vi "Create or Access Config Path.vi"(8 "error in":errorcluster, 10 "Check/Build Folders?":bool, 11 "Module Data":refnum<class "Rename.lvclass">) -> (0 "error out":errorcluster, 2 "Config File Path":path, 3 "Module Data":refnum<class "Rename.lvclass">)   [LabVIEW 2015, in "Generic Module Library.lvlib" / "Template G_Module.lvlib"]
uses:
  Template G_Module.lvlib
  <vilib>/Utility/sysdir.llb/System Directory Type.ctl
  Module Class/Rename.lvclass
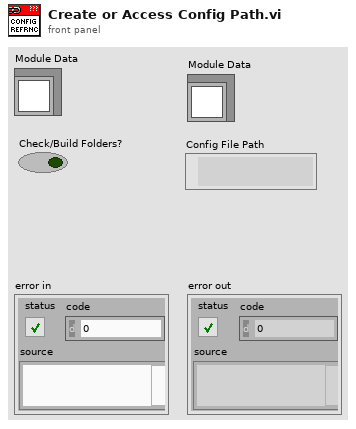
[diagram p1: front panel]
types:
  T1 = enum16{"open", "replace", "create", "open or create", "replace or create", "replace or create with confirmation"}
  T2 = typedef "System Directory Type.ctl" = i32
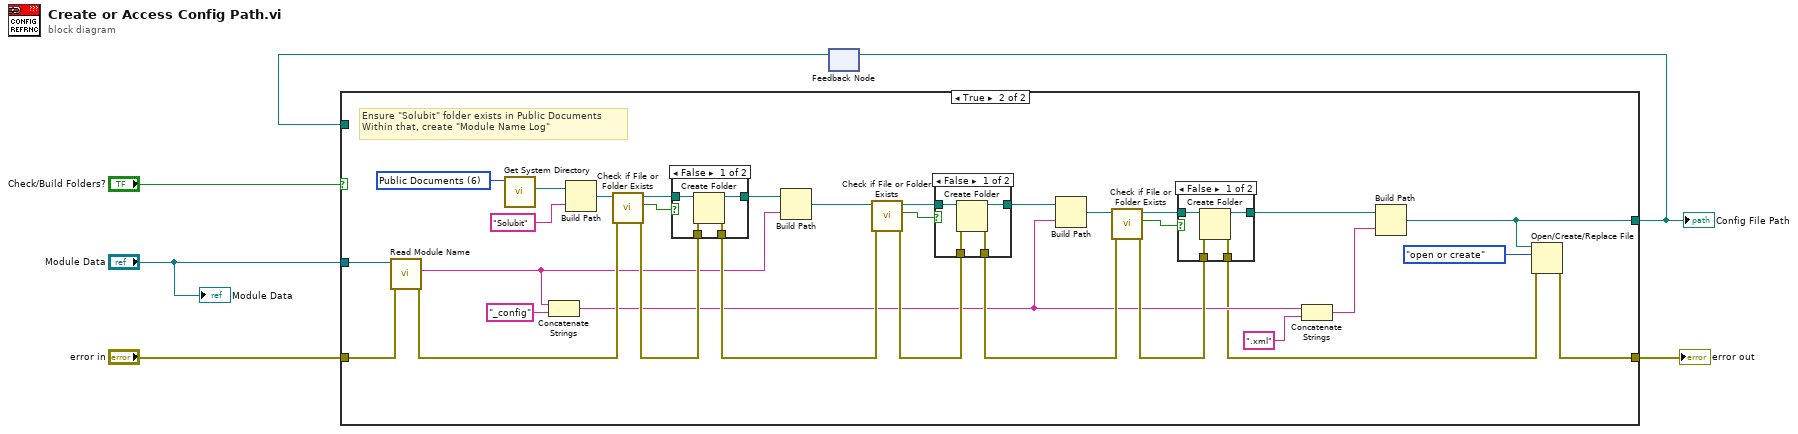
[diagram p0: block diagram]
diagram:
  n1 = feedback #1() -> (w2:path)  [unwired: 1 in]
  n2 = case shown="True" "Check/Build Folders?" {
    tunnel: "Module Data" -> [_ w33]
    tunnel: "error in" -> [w8 w32]
    tunnel: [w8 w10] -> w5
    tunnel: [w7 w12] -> w1
    tunnel: w2 -> [w7 _]
    frame False {
    }
    frame True {
      w40 = T2 6 items=["User Home"=0, "User Desktop"=1, "User Documents"=2, "User Application Data"=3, "User Preferences"=4, "User Temporary"=5, "Public Documents"=6, "Public Application Data"=7, "Public Preferences"=8, "Public Cache"=13, "System Core Libraries"=9, "System Installed Libraries"=10, "Application Files"=11, "Boot Volume Root"=12] ("system directory type")
      # "Ensure \"Solubit\" folder exists in Public Documents\nWithin that, create \"Module Name Log\""
      n3 = call-dynamic "Read Module Name.vi"("error in (no error)"=w32, "Rename in"=w33) -> ("error out"=w18:errorcluster, "Module Name"=w17:string)  [unwired: 7 in, 1 out]
      n4 = call <vilib>:"Get System Directory.vi"("system directory type"=w40) -> ("system directory"=w39:path)  [unwired: 10 in]
      n5 = Concatenate Strings(w17, "_config" ("string")) -> (w15:string)
      n6 = Build Path(base path=w39, name or relative path="Solubit") -> (appended path=w37:path)
      n7 = call <vilib>:"Check if File or Folder Exists.vi"("error in (no error)"=w18, "path"=w37) -> ("error out"=w34:errorcluster, "file or folder exists?"=w35:bool, "dup path"=w36:path)  [unwired: 7 in]
      n8 = case shown="False" w35 {
        tunnel: w36 -> [w50 w52]
        tunnel: w34 -> [w49 w51]
        tunnel: [w47 w51] -> w28
        tunnel: [w48 w52] -> w30
        frame False {
          n9 = Create Folder(path (use dialog)=w50, error in=w49) -> (created path=w48:path, error out=w47:errorcluster)  [unwired: 1 in, 1 out]
        }
        frame True {
        }
      }
      n10 = Build Path(base path=w30, name or relative path=w17) -> (appended path=w29:path)
      n11 = call <vilib>:"Check if File or Folder Exists.vi"("error in (no error)"=w28, "path"=w29) -> ("error out"=w25:errorcluster, "file or folder exists?"=w26:bool, "dup path"=w27:path)  [unwired: 7 in]
      n12 = case shown="False" w26 {
        tunnel: w27 -> [w44 w46]
        tunnel: w25 -> [w43 w45]
        tunnel: [w41 w45] -> w24
        tunnel: [w42 w46] -> w23
        frame False {
          n13 = Create Folder(path (use dialog)=w44, error in=w43) -> (created path=w42:path, error out=w41:errorcluster)  [unwired: 1 in, 1 out]
        }
        frame True {
        }
      }
      n14 = Build Path(base path=w23, name or relative path=w15) -> (appended path=w19:path)
      n15 = call <vilib>:"Check if File or Folder Exists.vi"("error in (no error)"=w24, "path"=w19) -> ("error out"=w20:errorcluster, "file or folder exists?"=w21:bool, "dup path"=w22:path)  [unwired: 7 in]
      n16 = case shown="False" w21 {
        tunnel: w22 -> [w56 w58]
        tunnel: w20 -> [w55 w57]
        tunnel: [w54 w57] -> w9
        tunnel: [w53 w58] -> w14
        frame False {
          n17 = Create Folder(path (use dialog)=w56, error in=w55) -> (created path=w53:path, error out=w54:errorcluster)  [unwired: 1 in, 1 out]
        }
        frame True {
        }
      }
      n18 = Concatenate Strings(w15, ".xml" ("string")) -> (w13:string)
      n19 = Build Path(base path=w14, name or relative path=w13) -> (appended path=w12:path)
      n20 = Open/Create/Replace File(file path (use dialog)=w12, error in=w9, operation (0:open)=T1."open or create") -> (error out=w10:errorcluster)  [unwired: 3 in, 2 out]
    }
  }
  "error out" <- w5
  "Config File Path" <- w1
  n21 = feedback-in #1(w1) -> ()
  "Module Data" <- "Module Data"
